vi "BeepMe.vi"(8 "error in (no error)":errorcluster, 9 "duration (3 msec)":u32=3, 10 "use system alert? (T)":bool, 11 "frequency (500 Hz)":u32=500) -> (0 "error out":errorcluster)   [LabVIEW 2013]
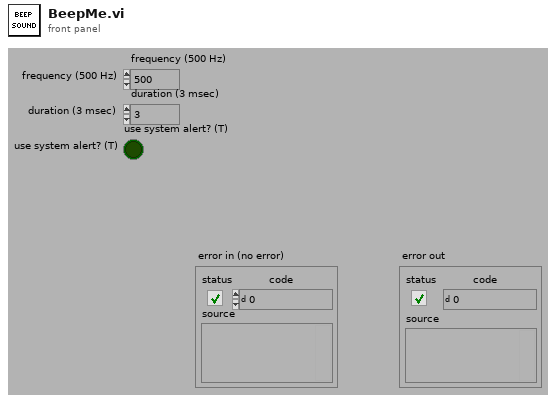
[diagram p1: front panel]
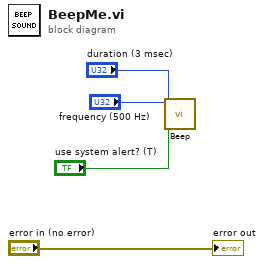
[diagram p0: block diagram]
diagram:
  n1 = call <vilib>:"Beep.vi"("use system alert? (T)"="use system alert? (T)", "duration (msec)"="duration (3 msec)", "frequency (Hz)"="frequency (500 Hz)") -> ()  [unwired: 9 in]
  "error out" <- "error in (no error)"
